vi "Return Aggregate Queues.vi"(11 "LoggerReference in":refnum<class "LoggerReference.lvclass">) -> (3 "Aggregate Loggers":refnum<queue>[](array[refnum]))   [LabVIEW 2020, in "Composed Log.lvlib" / "LoggerReference.lvclass"]
uses:
  <vilib>/gpm_packages/@cs/event-logger/Source/Composed Log/LoggerReference/LoggerReference.lvclass
  <vilib>/gpm_packages/@cs/event-logger/Source/Composed Log/Types/MessageCluster.ctl
  <vilib>/gpm_packages/@cs/event-logger/Source/Composed Log/LoggerReference/LoggerReference.lvclass/LoggerReference.ctl
  <vilib>/gpm_packages/@cs/event-logger/Source/Composed Log/Composed Log.lvlib
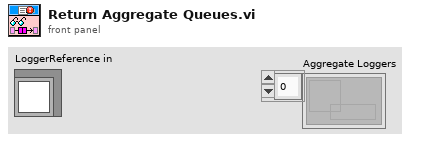
[diagram p1: front panel]
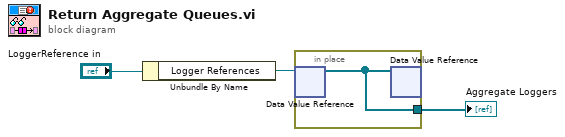
[diagram p0: block diagram]
diagram:
  n1 = Unbundle By Name("LoggerReference in") -> ("Logger References"=w2:refnum<data-value>)
  n2 = in-place {
    in-place-border: [w4] -> w1
    n3 = in-place-dvr #1(w2) -> (w4:refnum<queue>[])  [unwired: 1 out]
    n4 = in-place-dvr #1(w4) -> ()  [unwired: 2 out]
  }
  "Aggregate Loggers" <- w1
